vi "Check for Input.vi"(8 "error in (no error)":errorcluster, 9 "Control Refs":refnum<vi>[](array[refnum]), 10 "Mouse Ref":refnum<k1>, 11 "Step in":refnum<class "Step.lvclass">) -> (0 "error out":errorcluster, 3 "Step out":refnum<class "Step.lvclass">)   [LabVIEW 2020, in "MacroAssert.lvlib" / "Step.lvclass"]
uses:
  Step.lvclass
  Step.lvclass/Step.ctl
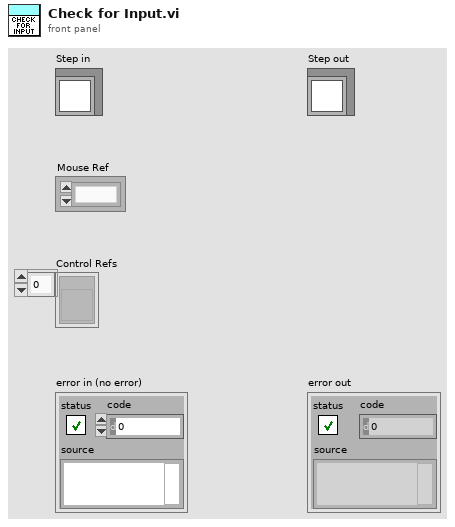
[diagram p1: front panel]
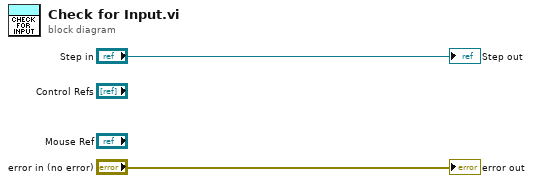
[diagram p0: block diagram]
diagram:
  "error out" <- "error in (no error)"
  "Step out" <- "Step in"
